vi "Parameters.vi"(8 "error in (no error)":errorcluster, 11 "Template Test Case In":refnum<class "Date Regex Finder Tests.lvclass">) -> (0 "error out":errorcluster, 2 "Parameters":T1(array[cluster]))   [LabVIEW 2020, in "Date Regex Finder Tests.lvclass"]
doc: "This VI defines the parameters used for execution. When LUnit runs the test case, it will run it once for every parameter in the array and collect the results.\n\nDuring test execution, the parameters are available in the class wire within the test VI."
uses:
  Date Regex Finder Tests.lvclass
  C:/Program Files/National Instruments/LabVIEW 2026/vi.lib/Astemes/LUnit Parameterized/Parameterized Test Case/Parameterized Test Case.lvclass
  <vilib>/Astemes/LUnit Parameterized/Parameterized Test Case/Parameterized Test Case.lvclass
  Parameters.ctl
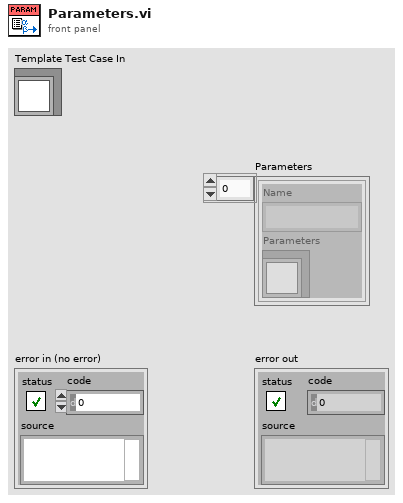
[diagram p1: front panel]
types:
  T1 = cluster{"Name":string, "Parameters":refnum<class "Parameterized Test Case.lvclass">}[]
  T2 = typedef "Date Regex Finder Tests.lvclass/Parameters.ctl" = cluster{"Date String":string, "Should Find? (T)":bool}
  T3 = cluster{"Scenario":string, "Parameters":refnum<class "Date Regex Finder Tests.lvclass">}[]
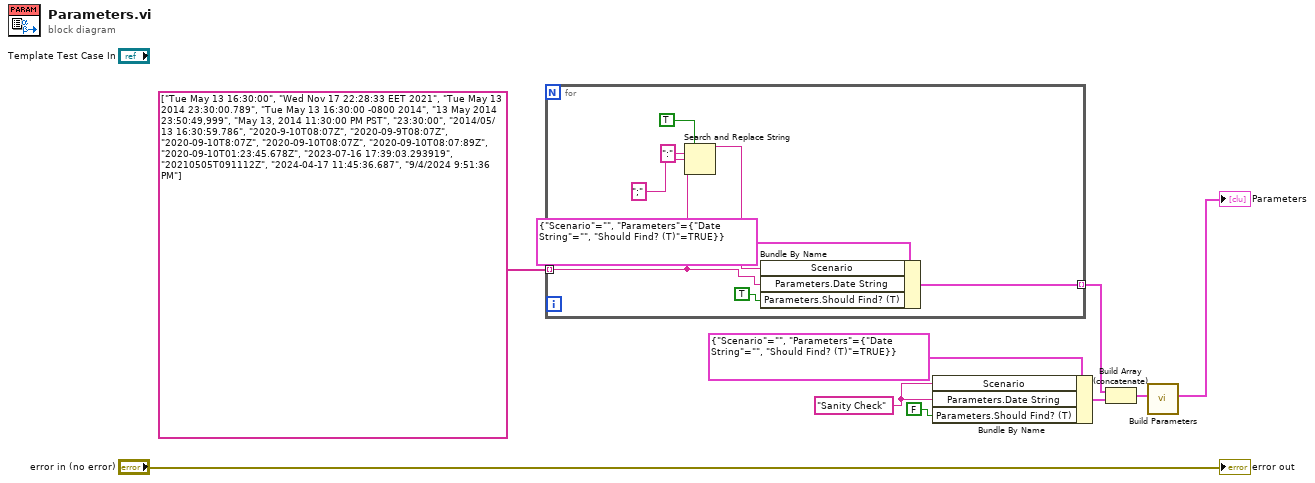
[diagram p0: block diagram]
diagram:
  w1 = "Sanity Check" ("Scenario")
  n1 = for {
    tunnel: string[] ["Tue May 13 16:30:00", "Wed Nov 17 22:28:33 EET 2021", "Tue May 13 2014 23:30:00.789", "Tue May 13 16:30:00 -0800 2014", "13 May 2014 23:50:49,999", "May 13, 2014 11:30:00 PM PST", "23:30:00", "2014/05/13 16:30:59.786", "2020-9-10T08:07Z", "2020-09-9T08:07Z", "2020-09-10T8:07Z", "2020-09-10T08:07Z", "2020-09-10T08:07:89Z", "2020-09-10T01:23:45.678Z", "2023-07-16 17:39:03.293919", "20210505T091112Z", "2024-04-17 11:45:36.687", "9/4/2024 9:51:36 PM"] ("subarray") -> [w14] mode=indexing
    tunnel: [w15] -> w4 mode=indexing
    n2 = Search and Replace String(replace all?=TRUE ("replace all? (F)"), input string=w14, search string=":", replace string=";" ("search string")) -> (result string=w11:string)  [unwired: 4 in, 3 out]
    n3 = Bundle By Name(cluster=cluster{"Scenario":string, "Parameters":T2} {"Scenario"="", "Parameters"={"Date String"="", "Should Find? (T)"=TRUE}}, "Scenario"=w11, "Parameters.Date String"=w14, "Parameters.Should Find? (T)"=TRUE) -> (w15:cluster{"Scenario":string, "Parameters":T2})
  }
  n4 = Bundle By Name(cluster=cluster{"Scenario":string, "Parameters":T2} {"Scenario"="", "Parameters"={"Date String"="", "Should Find? (T)"=TRUE}}, "Scenario"=w1, "Parameters.Date String"=w1, "Parameters.Should Find? (T)"=FALSE) -> (w3:cluster{"Scenario":string, "Parameters":T2})
  n5 = Build Array (concatenate)(w4, w3) -> (w2:cluster{"Scenario":string, "Parameters":T2}[])
  n6 = call "Build Parameters.vi"("Scenarios In"=w2) -> ("Scenarios out"=→"Parameters":T3)  [unwired: 10 in]
  "error out" <- "error in (no error)"
